vi "Try Parse.vi"(0 "SG 26GHz Path in":refnum<class "SG 26GHz Path.lvclass">, 5 "Config Row":string[](array[string]), 11 "error in":errorcluster) -> (4 "SG 26GHz Path out":refnum<class "SG 26GHz Path.lvclass">, 6 "Is of type?":bool, 15 "error out":errorcluster)   [LabVIEW 2023, in "RFFixtureCharact.PXI.lvlib" / "SG 26GHz Path.lvclass"]
uses:
  SG 26GHz Path.lvclass
  Common/RFCalAndFixtureCharact.Common.lvlib
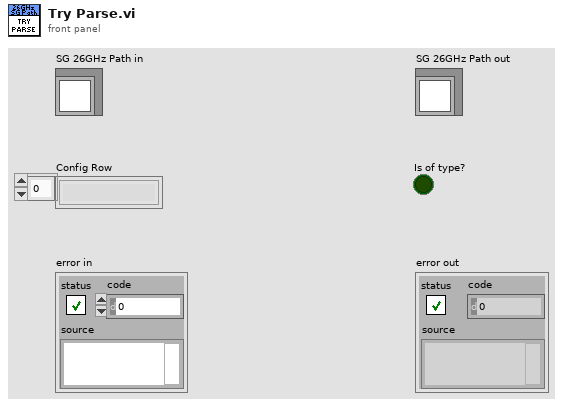
[diagram p1: front panel]
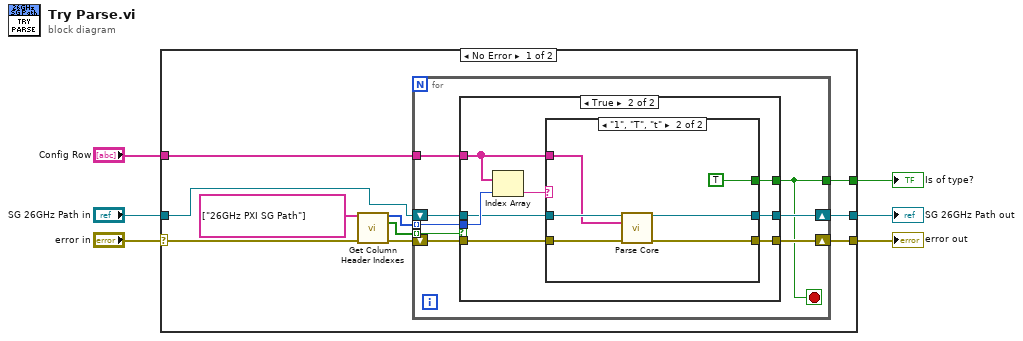
[diagram p0: block diagram]
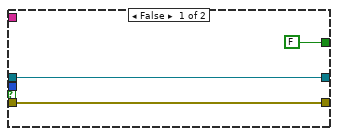
[diagram p2: hidden frame]
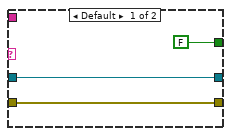
[diagram p3: hidden frame]
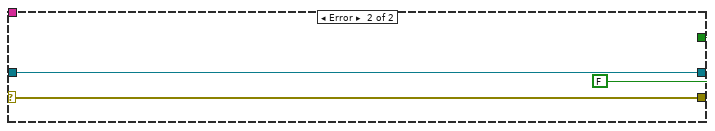
[diagram p4: hidden frame]
diagram:
  n1 = case shown="No Error" "error in" {
    selector: "error in" -> [w15 w47]
    tunnel: [w9 w47] -> w5
    tunnel: [w16 FALSE ("Is of type?")] -> w4
    tunnel: [w10 w46] -> w3
    tunnel: "Config Row" -> [w14 _]
    tunnel: "SG 26GHz Path in" -> [w8 w46]
    frame No Error {
      n2 = call "Get Column Header Indexes.vi"("Column Header Names"=string[] ["26GHz PXI SG Path"], "error in"=w15) -> ("Column Header Indices"=w11:i32[], "Column Header Exists?"=w7:bool[], "error out"=w13:errorcluster)  [unwired: 11 in]
      n3 = for {
        tunnel: [w18] -> w16
        tunnel: w14 -> [w24]
        tunnel: w11 -> [w22] mode=indexing
        shift-right: [w19] -> w9
        shift-left: w13 -> [w23]
        shift-right: [w20] -> w10
        shift-left: w8 -> [w21]
        tunnel: w7 -> [w17] mode=indexing
        stop <- w18 stop-if-true
        n4 = case shown="True" w17 {
          tunnel: [FALSE ("Is of type?") w35] -> w18
          tunnel: w24 -> [_ w34]
          tunnel: w23 -> [w26 w32]
          tunnel: w22 -> [_ w31]
          tunnel: w21 -> [w27 w30]
          tunnel: [w27 w29] -> w20
          tunnel: [w26 w28] -> w19
          frame False {
          }
          frame True {
            n5 = Index Array(array=w34, index=w31) -> (element=w33:string)
            n6 = case shown="\"1\", \"T\", \"t\"" w33 {
              tunnel: [w36 w44] -> w28
              tunnel: [FALSE ("Is of type?") TRUE ("Is of type?")] -> w35
              tunnel: [w38 w43] -> w29
              tunnel: w32 -> [w36 w42]
              tunnel: w30 -> [w38 w41]
              tunnel: w34 -> [_ w40]
              frame Default {
              }
              frame "1", "T", "t" {
                n7 = call-dynamic "Parse Core.vi"("Scalar Path in"=w41, "Config Row"=w40, "error in (no error)"=w42) -> ("Scalar Path out"=w43:refnum<class "SG 26GHz Path.lvclass">, "error out"=w44:errorcluster)  [unwired: 11 in]
              }
            }
          }
        }
      }
    }
    frame Error {
    }
  }
  "error out" <- w5
  "SG 26GHz Path out" <- w3
  "Is of type?" <- w4
